vi "LowPass.vi"() -> ()   [LabVIEW 2011]
doc: "This example demonstrates how to use the IIR Cascade Filter VI to perform online filtering without having to compensate for the initial transient after the first block of data is filtered.\n\nThis example repeatedly generates a noisy sinewave and filters it using two different methods. \n\nThe first method uses the memory mechanism of the IIR Cascade Filter VI to retain state information about previous inputs and outputs of the filter in order to eliminate the transient. \n\nThe second method uses no memory mechanism causing the IIR Cascade Filter VI to assume zero initial conditions each time the VI is called. The result is that on each iteration this method produces a transient rather than the filtered signal."
uses:
  <vilib>/Analysis/baseanly.llb/IIR Cascade Filter (DBL).vi
  <vilib>/Analysis/NI_AALBase.lvlib
panel:
  in  "Type of Graph":u16(ring)
  out "Waveform Graph 2":dbl[](graph)
  out "Waveform Graph":dynamicdata(graph)
  in  "stop":bool
  # "IIR CASCADE FILTER PROGRAM"
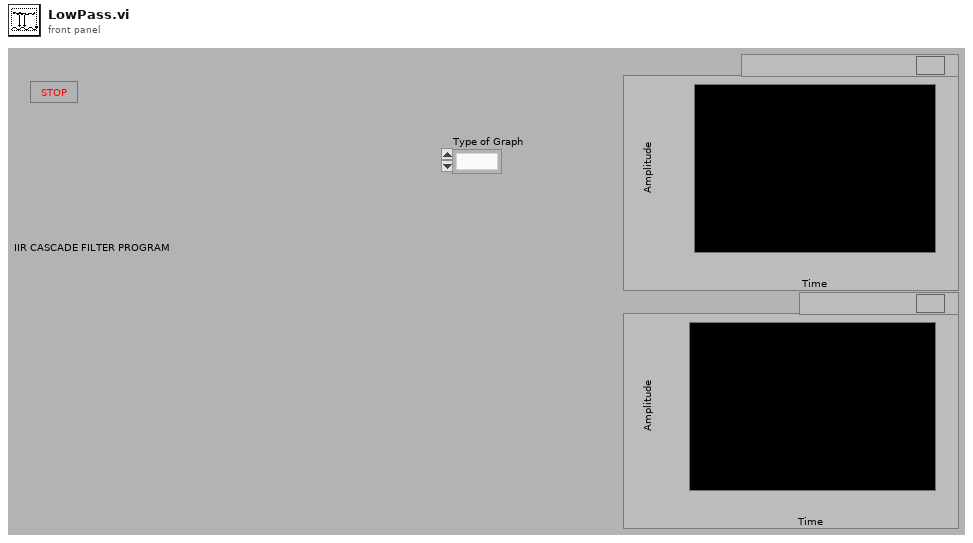
[diagram p1: front panel]
types:
  T1 = cluster{"filter structure":enum32{"IIR 2nd Order", "IIR 4th Order"}, "Reverse Coefficients":dbl[], "Forward Coefficients":dbl[]}
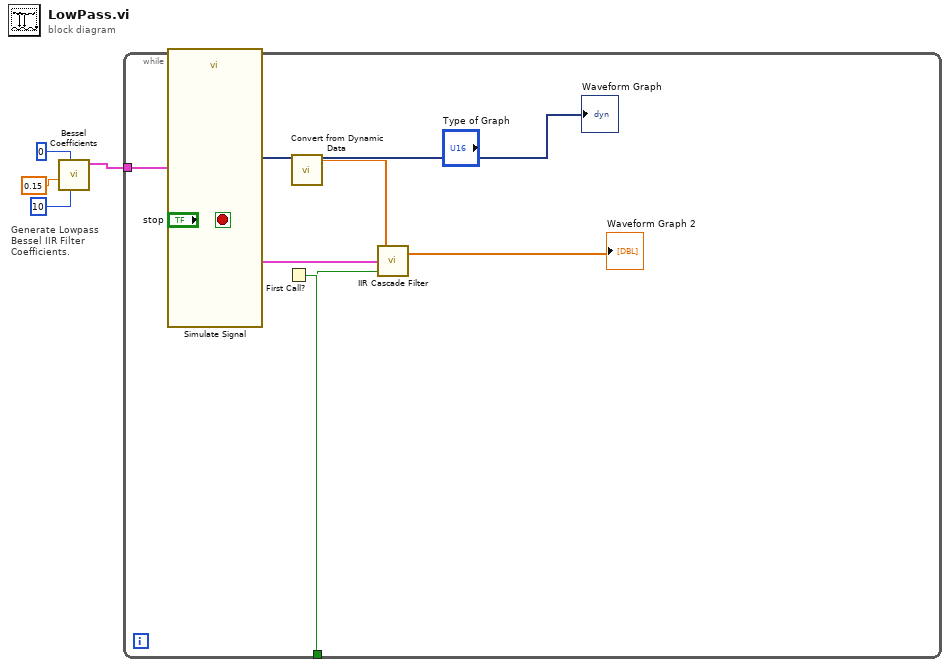
[diagram p0: block diagram]
diagram:
  # "Generate Lowpass\nBessel IIR Filter \nCoefficients."
  n1 = call <vilib>:"Bessel Coefficients.vi"("order"=10, "filter type"=0, "low cutoff freq: fl"=0.15) -> ("IIR Filter Cluster"=w4:T1)  [unwired: 7 in, 1 out]
  n2 = First Call?() -> (First Call?: T/F=w1:bool)
  n3 = while {
    tunnel: w4 -> [w11]
    tunnel: w1 -> [w9]
    stop <- "stop" stop-if-true
    n4 = call "Simulate Signal"() -> ("Triangle with Inverse F Noise"=w8:dynamicdata)  [unwired: 14 in, 1 out]
    "Waveform Graph" <- w8
    n5 = call "Convert from Dynamic Data"("Dynamic Data Type"=w8) -> ("Array"=w7:dbl[])  [unwired: 3 in]
    n6 = call-poly <vilib>:"IIR Cascade Filter.vi"("init/cont (init:F)"=w9, "IIR Filter Cluster"=w11, "X"=w7) -> ("Filtered X"=→"Waveform Graph 2":dbl[])  [unwired: 1 out]
  }
